vi "Merge_valid_row_values.vi"(3 "Present Row values":string[](array[string]), 4 "Present Channels":string[](array[string]), 5 "Desired Channels":string[](array[string])) -> (0 "Merged?":bool, 1 "Achieved Row values":string[](array[string]), 2 "Achieved Channels":string[](array[string]))   [LabVIEW 2010]
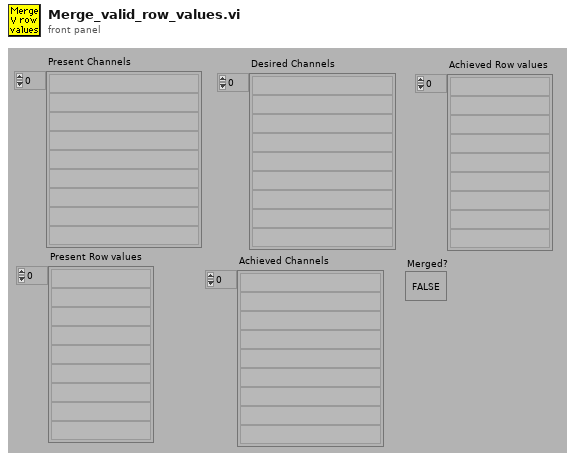
[diagram p1: front panel]
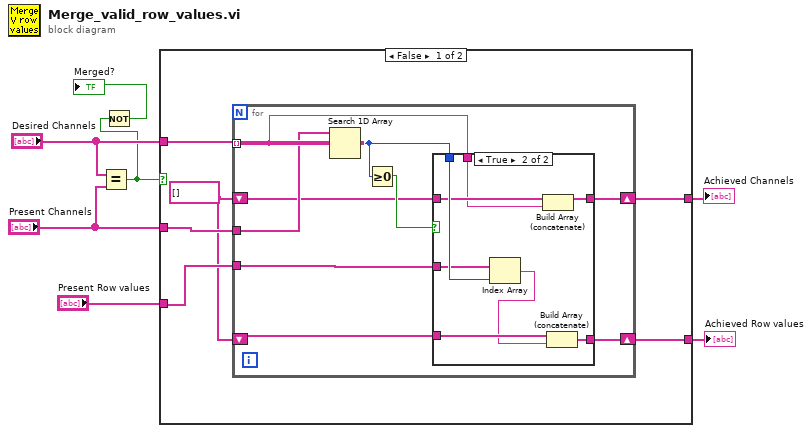
[diagram p0: block diagram]
diagram:
  n1 = Equal?(x="Desired Channels", y="Present Channels") -> (x = y?=w3:bool)
  n2 = Not(x=w3) -> (.not. x?=→"Merged?":bool)
  n3 = case shown="False" w3 {
    tunnel: "Present Channels" -> [w13 _]
    tunnel: "Desired Channels" -> [w12 w33]
    tunnel: [w8 w34] -> w5
    tunnel: "Present Row values" -> [w11 w34]
    tunnel: [w9 w33] -> w1
    frame False {
      w10 = string[] []
      n4 = for {
        tunnel: w13 -> [w22]
        tunnel: w12 -> [w17] mode=indexing
        tunnel: w11 -> [w21]
        shift-right: [w16] -> w9
        shift-left: w10 -> [w18]
        shift-right: [w14] -> w8
        shift-left: w10 -> [w15]
        n5 = Search 1D Array(1D array=w22, element=w17) -> (index of element=w20:i32)  [unwired: 1 in]
        n6 = Greater Or Equal To 0?(x=w20) -> (x >= 0?=w19:bool)
        n7 = case shown="True" w19 {
          tunnel: w20 -> [_ w32]
          tunnel: w21 -> [_ w31]
          tunnel: w18 -> [w24 w30]
          tunnel: w17 -> [_ w29]
          tunnel: [w24 w28] -> w16
          tunnel: w15 -> [w23 w27]
          tunnel: [w23 w26] -> w14
          frame False {
          }
          frame True {
            n8 = Index Array(array=w31, index=w32) -> (element=w25:string)
            n9 = Build Array (concatenate)(w30, w29) -> (w28:string[])
            n10 = Build Array (concatenate)(w27, w25) -> (w26:string[])
          }
        }
      }
    }
    frame True {
    }
  }
  "Achieved Row values" <- w5
  "Achieved Channels" <- w1
